vi "Add Custom Device.vi"(8 "error in":errorcluster, 10 "name":string, 11 "target in":refnum<k24>) -> (0 "error out":errorcluster, 2 "custom device":T1 format="%.0x", 3 "target out":refnum<k24>)   [LabVIEW 2025, in "AIM ARINC 664 Scripting.lvlib"]
doc: "Adds the AIM ARINC 664 custom device to the system definition. Required sections for <b>Configuration Files</b>, <b>Ports</b> and <b>Status</b> are added within the custom device. Returns the newly added <b>custom device</b> reference."
uses:
  AIM ARINC 664 Scripting.lvlib
  NationalInstruments.VeriStand.SystemDefinitionAPI
  <vilib>/NI VeriStand/Custom Device Tools/Custom Device Utility Library/Custom Device Utility Library.lvlib
  <vilib>/NI VeriStand/Custom Device API/Custom Device Item Ref.ctl
  <vilib>/NI VeriStand/Custom Device API/Custom Device API.lvlib
  Constants.vi
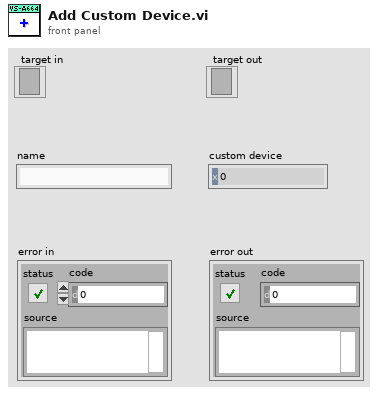
[diagram p1: front panel]
types:
  T1 = typedef "Custom Device API.lvlib/Custom Device Item Ref.ctl" = u64
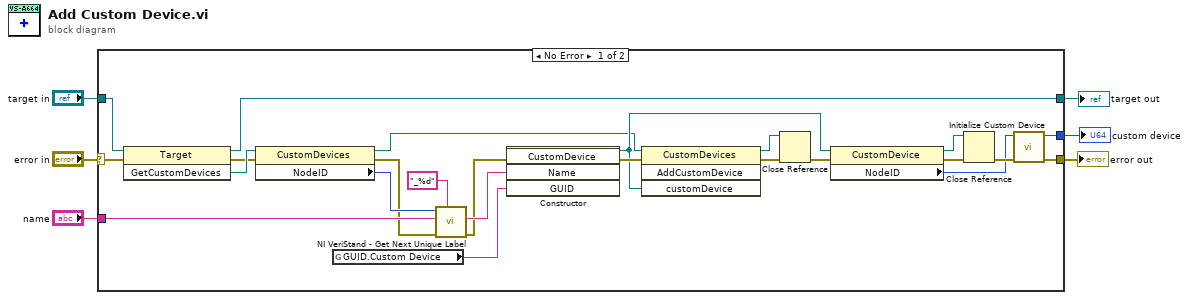
[diagram p0: block diagram]
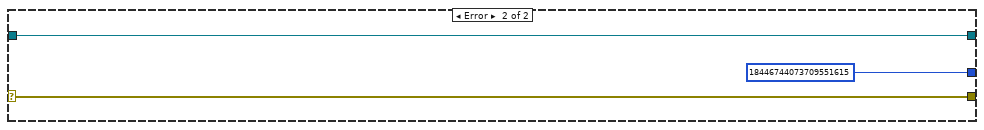
[diagram p2: hidden frame]
diagram:
  n1 = case shown="No Error" "error in" {
    selector: "error in" -> [w29 w33]
    tunnel: "target in" -> [w30 w32]
    tunnel: [w7 w33] -> w4
    tunnel: "name" -> [w17 _]
    tunnel: [w8 T1 18446744073709551615 ("Custom device Ref out")] -> w2
    tunnel: [w21 w32] -> w1
    frame No Error {
      n2 = invoke on="Invoke Node" class="Target" method="GetCustomDevices"(reference=w30, error in=w29) -> (reference out=w21:refnum<k24>, error out=w14:errorcluster, "GetCustomDevices"=w19:refnum<k24>)  [unwired: 1 in]
      n3 = property on="Property Node" class="CustomDevices"(reference=w19, error in=w14) -> (reference out=w13:refnum<k24>, error out=w12:errorcluster, "NodeID"=w18:u64)
      n4 = global read "Constants.vi" "GUID.Custom Device"() -> (w20:string)
      n5 = call <vilib>:"NI VeriStand - Get Next Unique Label.vi"("format string"="_%d", "error in (no error)"=w12, "Label"=w17, "Parent Ref in"=w18) -> ("error out"=w11:errorcluster, "Label out"=w15:string)  [unwired: 4 in, 2 out]
      n6 = constructor class="CustomDevice" ("Constructor Node")(error in=w11, "Name"=w15, "GUID"=w20) -> (reference out=w25:refnum<k24>, error out=w28:errorcluster)  [unwired: 2 in, 3 out]
      n7 = invoke on="Invoke Node" class="CustomDevices" method="AddCustomDevice"(reference=w13, error in=w28, "customDevice"=w25) -> (reference out=w22:refnum<k24>, error out=w24:errorcluster)  [unwired: 1 in, 2 out]
      n8 = Close Reference(reference=w22, error in (no error)=w24) -> (error out=w23:errorcluster)
      n9 = property on="Property Node" class="CustomDevice"(reference=w25, error in=w23) -> (reference out=w27:refnum<k24>, error out=w26:errorcluster, "NodeID"=w9:u64)
      n10 = Close Reference(reference=w27, error in (no error)=w26) -> (error out=w10:errorcluster)
      n11 = call "Initialize Custom Device.vi"("error in"=w10, "custom device ref"=w9) -> ("error out"=w7:errorcluster, "custom device ref out"=w8:T1)  [unwired: 8 in]
    }
    frame Error {
    }
  }
  "error out" <- w4
  "custom device" <- w2
  "target out" <- w1
